vi "Write Text.vi"(8 "error in (no error)":errorcluster, 9 "Data":string, 10 "timeout ms (5000)":i32=5000, 11 "RawSocket Handler in":refnum<class "RawSocket TCP Handler.lvclass">) -> (0 "error out":errorcluster, 3 "RawSocket Handler out":refnum<class "RawSocket TCP Handler.lvclass">)   [LabVIEW 2020, in "wamplv.lvlib" / "RawSocket TCP Handler.lvclass"]
uses:
  RawSocket TCP Handler.lvclass
  RawSocket TCP Handler.lvclass/RawSocket TCP Handler.ctl
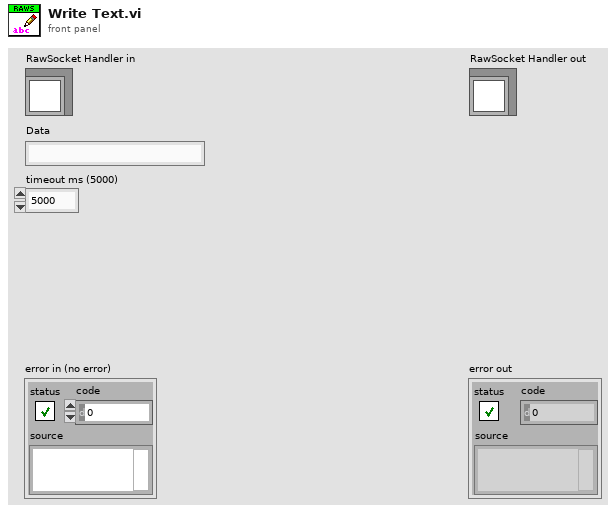
[diagram p1: front panel]
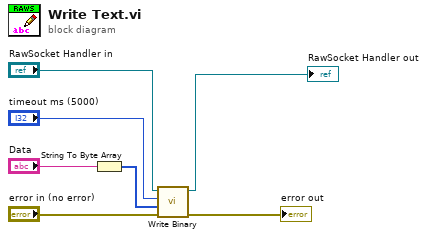
[diagram p0: block diagram]
diagram:
  n1 = String To Byte Array(string="Data") -> (unsigned byte array=w2:u8[])
  n2 = call-dynamic "Write Binary.vi"("error in (no error)"="error in (no error)", "Bytes"=w2, "timeout ms (5000)"="timeout ms (5000)", "RawSocket TCP Handler in"="RawSocket Handler in") -> ("error out"=→"error out":errorcluster, "RawSocket TCP Handler out"=→"RawSocket Handler out":refnum<class "RawSocket TCP Handler.lvclass">)  [unwired: 4 in]
